vi "IsEnabled.vi"(8 "error in (no error)":errorcluster, 11 "FHPP in":refnum<class "FHPP.lvclass">) -> (0 "error out":errorcluster, 1 "Operation Enabled":bool, 2 "Drive Enabled":bool, 3 "FHPP out":refnum<class "FHPP.lvclass">)   [LabVIEW 2022 SP3, in "FHPP.lvclass"]
uses:
  FHPP.lvclass
  FHPP.lvclass/FHPP.ctl
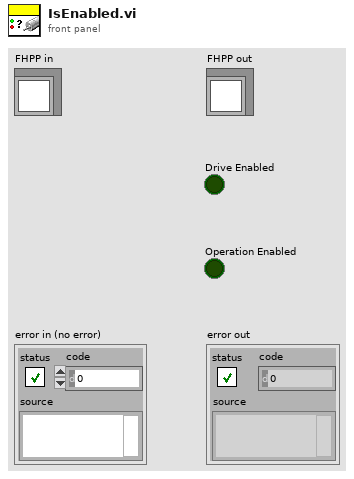
[diagram p1: front panel]
types:
  T1 = typedef "FHPP.lvclass/SCON.ctl" = cluster{"Drive Enabled":bool, "Operation Enabled":bool, "Warning":bool, "Error":bool, "Load Voltage Applied":bool, "FCT/MMI":bool, "Operation Mode":T2}
  T2 = typedef "FHPP.lvclass/Operating Mode.ctl" = enum16{"Record Selection", "Direct Mode", "Reserved 1", "Reserved 2"}
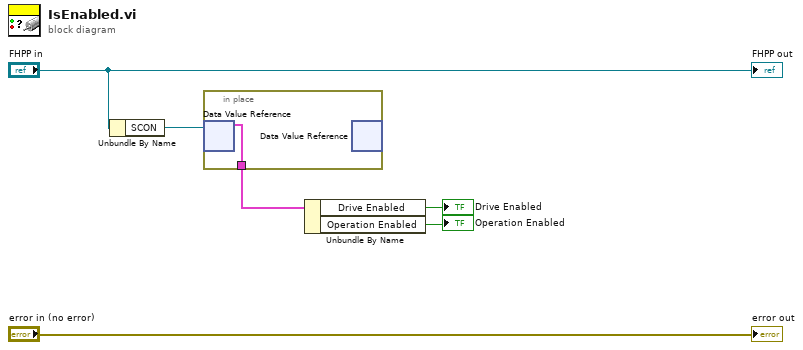
[diagram p0: block diagram]
diagram:
  n1 = Unbundle By Name("FHPP in") -> ("SCON"=w4:refnum<data-value>)
  n2 = in-place {
    in-place-border: [w7] -> w3
    n3 = in-place-dvr #1(w4) -> (w7:T1)  [unwired: 1 out]
    n4 = in-place-dvr #1() -> ()  [unwired: 1 in, 2 out]
  }
  n5 = Unbundle By Name(w3) -> ("Drive Enabled"=→"Drive Enabled":bool, "Operation Enabled"=→"Operation Enabled":bool)
  "error out" <- "error in (no error)"
  "FHPP out" <- "FHPP in"
